vi "Launcher.vi"   [LabVIEW 2020]
uses:
  <vilib>/MGI/Panel Manager/Panel/Window Position/Reference Position/Alignment.ctl
  <vilib>/MGI/Panel Manager/Panel/Window Position/Reference Position/Horizontal Alignment.ctl
  <vilib>/MGI/Panel Manager/Panel/Window Position/Reference Position/Vertical Alignment.ctl
  GUI.lvclass
  C:/Program Files/National Instruments/LabVIEW 2020/vi.lib/MGI/Panel Manager/Panel Actor/Panel Actor/Panel Actor.lvclass
  <vilib>/MGI/Panel Manager/Panel/Window Position/Reference Position/Offset/Absolute Offset/Absolute Offset.vi
  <vilib>/MGI/Panel Manager/Panel/Window Position/Reference Position/Ref VI/Ref VI.lvclass
  C:/Program Files/National Instruments/LabVIEW 2020/vi.lib/MGI/Panel Manager/Panel/Window Position/Window Position.lvclass
  <vilib>/MGI/Panel Manager/Panel/Window Position/Reference Position/Ref VI/Ref VI.vi
  <vilib>/MGI/Panel Manager/Panel Actor/Panel Actor/Launch Root Panel Window.vi
  <vilib>/MGI/Panel Manager/Panel/Window Position/Reference Position/Offset/Absolute Offset/Absolute Offset.lvclass
  <vilib>/MGI/Panel Manager/Panel Actor/Panel Actor/Panel Actor.lvclass
  <vilib>/MGI/Panel Manager/Panel/Panel.lvlib
  <vilib>/MGI/Panel Manager/Panel/Window Position/Reference Position/Reference Position.lvclass
  C:/Program Files/National Instruments/LabVIEW 2020/vi.lib/MGI/Panel Manager/Panel/Window Position/Reference Position/Reference Position.lvclass
  C:/Program Files/National Instruments/LabVIEW 2020/vi.lib/MGI/Panel Manager/Panel/Window Position/Reference Position/Ref VI/Ref VI.lvclass
  C:/Program Files/National Instruments/LabVIEW 2020/vi.lib/MGI/Monitored Actor/Monitored Actor/Monitored Actor/Monitored Actor.lvclass
  C:/Program Files/National Instruments/LabVIEW 2020/vi.lib/ActorFramework/Actor/Actor.lvclass
  W:/Parabolic Flight Bimanual/Labview Code/Bim Coord Local/GUI/GUI.lvclass
  W:/Parabolic Flight Bimanual/Labview Code/Bim Coord Local/GUI Interface/GUI Interface.lvclass
types:
  T1 = typedef "Panel.lvlib/Reference Position.lvclass/Alignment.ctl" = cluster{"Horizontal":T2, "Vertical":T3}
  T2 = typedef "Panel.lvlib/Reference Position.lvclass/Horizontal Alignment.ctl" = enum16{"Left", "Center", "Right"}
  T3 = typedef "Panel.lvlib/Reference Position.lvclass/Vertical Alignment.ctl" = enum16{"Top", "Center", "Bottom"}
  T4 = typedef "LVRectTypeDef.ctl" = cluster{"Left":i16, "Top":i16, "Right":i16, "Bottom":i16}
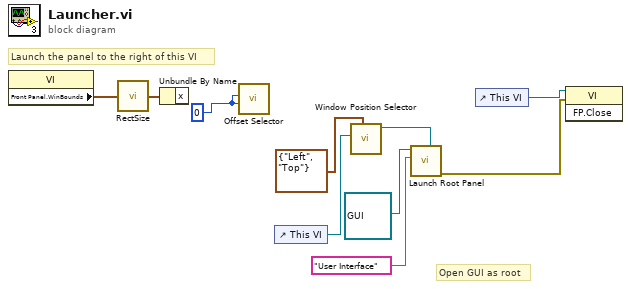
[diagram p0: block diagram]
diagram:
  w1 = i16 0 ("Horizontal")
  # "Open GUI as root"
  # "Launch the panel to the right of this VI"
  n1 = property class="VI"() -> ("Front Panel.WinBounds"=w6:T4)  [unwired: 2 in, 2 out]
  n2 = call <vilib>:"RectSize.vi"("rect"=w6) -> ("point"=w5:cluster{"x":i16, "y":i16})
  n3 = Unbundle By Name(w5) -> ()  [unwired: 1 out]
  n4 = call-poly <vilib>:"Offset Selector.vi"("Vertical"=w1, "Horizontal"=w1) -> ()  [unwired: 8 in, 2 out]
  n5 = control-ref of="This VI"() -> (w7:refnum<vi>)
  n6 = call-poly <vilib>:"Window Position Selector.vi"("Alignment"=T1 {"Horizontal"=enum."Left", "Vertical"=enum."Top"}, "Ref VI"=w7) -> ("Ref VI out"=w9:refnum<class "Ref VI.lvclass">)  [unwired: 8 in, 1 out]
  n7 = call-poly <vilib>:"Launch Root Panel.vi"("Window Position (Maximize First Call)"=w9, "Title"="User Interface", "Panel Actor in"=refnum<class "GUI.lvclass"> refnum ("GUI.lvlib:GUI.lvclass")) -> ("Error Out"=w2:errorcluster)  [unwired: 7 in, 1 out]
  n8 = control-ref of="This VI"() -> (w3:refnum<vi>)
  n9 = invoke class="VI" method="FP.Close"(reference=w3, error in=w2) -> ()  [unwired: 1 in, 3 out]
